vi "BuildVIP.vi"   [LabVIEW 2021]
uses:
  <vilib>/Wiresmith Technology/G CLI/CLI Class/CLI.lvclass
  <vilib>/JKI/VIPM API/VIPM API_vipm_api.lvlib
types:
  T1 = enum32{"Invalid", "Standard", "Closed", "Hidden", "Minimized", "Maximized"}
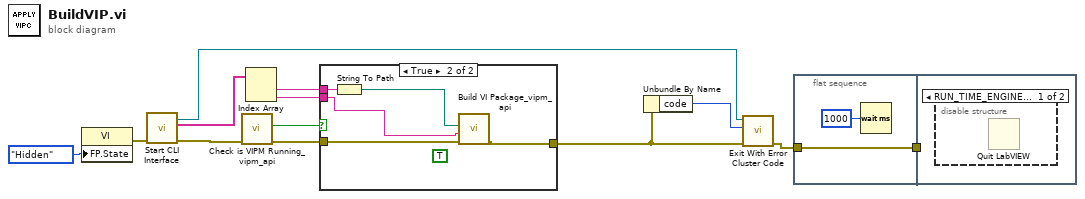
[diagram p0: block diagram]
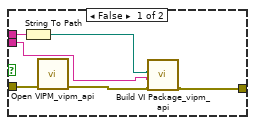
[diagram p3: hidden frame]
diagram:
  n1 = property class="VI"("FP.State"=T1."Hidden" ("Front Panel Window:State")) -> (error out=w12:errorcluster)  [unwired: 2 in, 1 out]
  n2 = call <vilib>:"Start CLI Interface.vi"("error in (no error)"=w12) -> ("error out"=w2:errorcluster, "Custom Parameters"=w8:string[], "CLI out"=w11:refnum<class "CLI.lvclass">)  [unwired: 7 in, 1 out]
  n3 = call <vilib>:"Check is VIPM Running_vipm_api.vi"("error in (no error)"=w2) -> ("error out"=w10:errorcluster, "is Running"=w9:bool)  [unwired: 9 in]
  n4 = Index Array(array=w8) -> (element #1=w3:string, element #2=w1:string)  [unwired: 2 in]
  n5 = case shown="True" w9 {
    tunnel: w10 -> [w19 w22]
    tunnel: w3 -> [w18 w24]
    tunnel: [w17 w23] -> w4
    tunnel: w1 -> [w14 w20]
    frame False {
      n6 = String To Path(string=w18) -> (path=w15:path)
      n7 = call <vilib>:"Open VIPM_vipm_api.vi"("error in (no error)"=w19) -> ("error out"=w16:errorcluster)  [unwired: 10 in]
      n8 = call <vilib>:"Build VI Package_vipm_api.vi"("error in (no error)"=w16, "LabVIEW Version"=w14, "Path to VIPB File"=w15) -> ("error out"=w17:errorcluster)  [unwired: 7 in, 1 out]
    }
    frame True {
      (unwired) TRUE ("quiet? (T)")
      n9 = String To Path(string=w24) -> (path=w21:path)
      n10 = call <vilib>:"Build VI Package_vipm_api.vi"("error in (no error)"=w22, "LabVIEW Version"=w20, "Path to VIPB File"=w21) -> ("error out"=w23:errorcluster)  [unwired: 7 in, 1 out]
    }
  }
  n11 = Unbundle By Name(w4) -> ("code"=w5:i32)
  n12 = call <vilib>:"Exit With Error Cluster Code.vi"("error in (no error)"=w4, "No Error Code (0)"=w5, "CLI in"=w11) -> ("error out"=w6:errorcluster)  [unwired: 8 in]
  n13 = flat-sequence {
    tunnel: w6 -> [w26]
    tunnel: [w26] -> w7
    tunnel: w7 -> [_]
    frame #0 {
      n14 = Wait (ms)(milliseconds to wait=u32 1000) -> ()  [unwired: 1 out]
    }
    frame #1 {
      n15 = disable-structure shown="RUN_TIME_ENGINE==True" {
        frame condition #0 {
          n16 = Quit LabVIEW() -> ()  [unwired: 1 in]
        }
        frame condition #1 (active) {
        }
      }
    }
  }
